vi "1 逻辑运算实现温度报警器.vi"() -> ()   [LabVIEW 2019]
panel:
  out "当前所测温度":dbl
  out "温度计":dbl(slide) scale=0.0..100.0
  in  "温度":dbl
  out "温度正常":bool
  out "温度过低":bool
  out "温度过高":bool
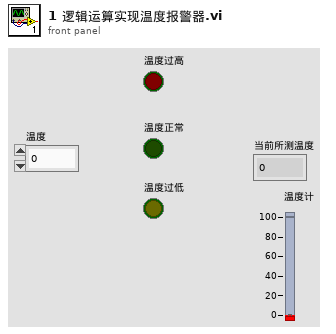
[diagram p1: front panel]
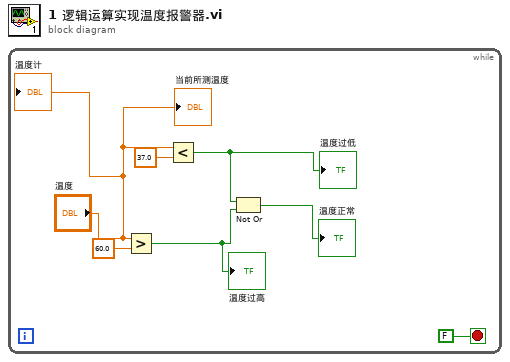
[diagram p0: block diagram]
diagram:
  n1 = while {
    stop <- FALSE stop-if-true
    n2 = Greater?(x="温度", y=60.0) -> (0:w4:bool)
    "温度过高" <- w4
    n3 = Less?(x="温度", y=37.0) -> (x < y?=w3:bool)
    "温度过低" <- w3
    n4 = Not Or(1:w4, 2:w3) -> (0:→"温度正常":bool)
    "温度计" <- "温度"
    "当前所测温度" <- "温度"
  }
